vi "Constants.vi"() -> ()   [LabVIEW 2016, in "Async UDP Shared.lvlib"]
doc: "Use this Global VI to access the GUIDs assigned to the page resources of the Custom Device."
uses:
  Async UDP Shared.lvlib
panel:
  in  "Tab Control":enum32{"GUIDS", "Constants", "Properties"}(tab)=enum."Constants"
  in  "Async UDP":string="00ed0b96-e65e-43f0-8de8-3523c97589e6"
  in  "UDP Remote Port":string="UDP Remote Port"
  in  "Address":string="Address"
  in  "UDP Local Port":string="UDP Local Port"
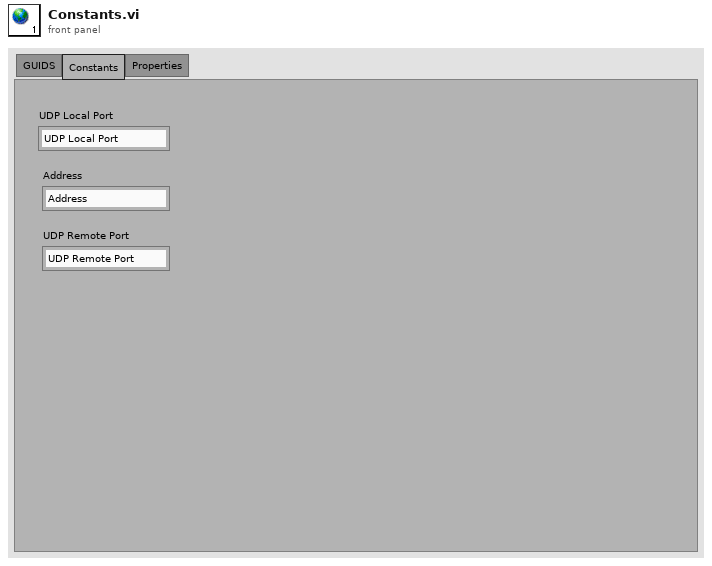
[diagram p1: front panel]
diagram:
